vi "Get All Sub-vis in Heirarchy.vi"(8 "error in (no error)":errorcluster, 11 "Start Vi":refnum<vi>) -> (0 "error out":errorcluster, 2 "All sub-vi nodes in heirarchy":refnum<vi>[](array[refnum]), 3 "Start Vi out":refnum<vi>, 4 "Vi Names":string[](array[string]), 5 "Vi-Refs":refnum<vi>[](array[refnum]))   [LabVIEW 2012, in "Scripting Tools.lvlib"]
doc: "Returns all the sub-vi nodes in all the diagrams of all the vis in the heirarchy, starting from <b>Start Vi</b>. Also returns a list of references to the vis (as opposed to the sub-vi nodes) and to the vi names."
uses:
  Scripting Tools.lvlib
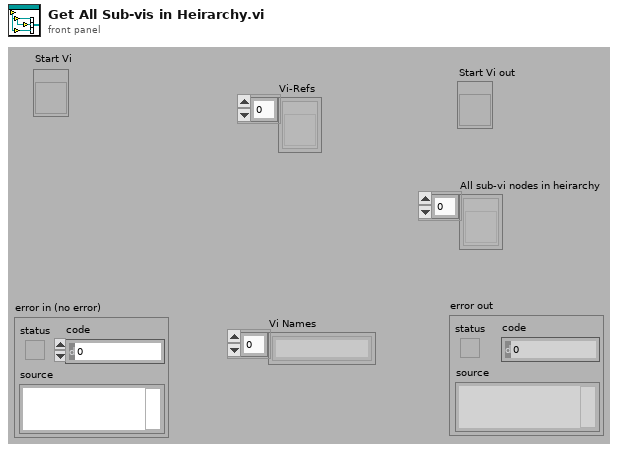
[diagram p1: front panel]
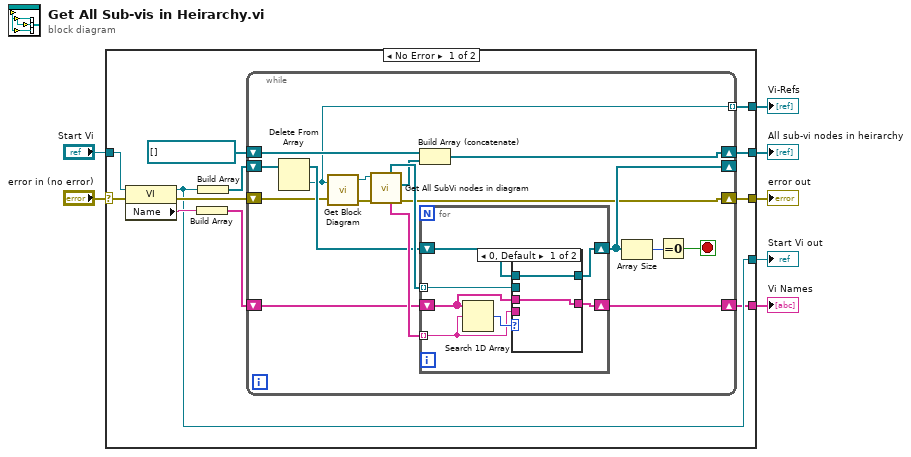
[diagram p0: block diagram]
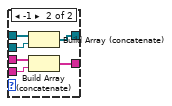
[diagram p2: hidden frame]
diagram:
  n1 = case shown="No Error" "error in (no error)" {
    selector: "error in (no error)" -> [w11 w53]
    tunnel: "Start Vi" -> [w17 w52]
    tunnel: [w14 _] -> w6
    tunnel: [w12 w53] -> w5
    tunnel: [w10 w52] -> w3
    tunnel: [w9 _] -> w2
    tunnel: [w8 _] -> w1
    frame No Error {
      n2 = property class="VI"(reference=w17, error in=w11) -> (reference out=w10:refnum<vi>, error out=w13:errorcluster, "Name"=w16:string)
      n3 = Build Array(w16) -> (w18:string[])
      n4 = Build Array(w10) -> (w19:refnum<vi>[])
      n5 = while {
        shift-right: [w24] -> w14
        shift-left: refnum<vi>[] [] -> [w23]
        shift-right: [w28] -> _
        shift-left: w19 -> [w36]
        shift-right: [w29] -> w8
        shift-left: w18 -> [w31]
        shift-right: [w21] -> w12
        shift-left: w13 -> [w22]
        tunnel: [w20] -> w9 mode=indexing
        stop <- w26 stop-if-true
        n6 = Delete From Array(array=w36) -> (deleted portion=w20:refnum<vi>, array with subset deleted=w30:refnum<vi>[])  [unwired: 2 in]
        n7 = call "Get Block Diagram.vi"("vi refnum in"=w20, "error in (no error)"=w22) -> ("Diagram"=w35:refnum<vi>, "error out"=w34:errorcluster)  [unwired: 1 out]
        n8 = call "Get All SubVi nodes in diagram.vi"("error in"=w34, "Diagram In"=w35) -> ("error out"=w21:errorcluster, "All Sub-vis"=w25:refnum<vi>[], "Vi Names"=w32:string[], "Vi-Refs"=w33:refnum<vi>[])  [unwired: 6 out]
        n9 = Build Array (concatenate)(w23, w25) -> (w24:refnum<vi>[])
        n10 = for {
          tunnel: w33 -> [w37] mode=indexing
          tunnel: w32 -> [w41] mode=indexing
          shift-right: [w40] -> w29
          shift-left: w31 -> [w42]
          shift-right: [w38] -> w28
          shift-left: w30 -> [w39]
          n11 = Search 1D Array(1D array=w42, element=w41) -> (index of element=w43:i32)  [unwired: 1 out]
          n12 = case shown="0, Default" w43 {
            tunnel: w42 -> [w45 w49]
            tunnel: w41 -> [_ w51]
            tunnel: [w45 w50] -> w40
            tunnel: w39 -> [w44 w48]
            tunnel: [w44 w47] -> w38
            tunnel: w37 -> [_ w46]
            frame 0, Default {
            }
            frame -1 {
              n13 = Build Array (concatenate)(w48, w46) -> (w47:refnum<vi>[])
              n14 = Build Array (concatenate)(w49, w51) -> (w50:string[])
            }
          }
        }
        n15 = Array Size(array=w28) -> (size(s)=w27:i32)
        n16 = Equal To 0?(x=w27) -> (x = 0?=w26:bool)
      }
    }
    frame Error {
    }
  }
  "All sub-vi nodes in heirarchy" <- w6
  "error out" <- w5
  "Start Vi out" <- w3
  "Vi-Refs" <- w2
  "Vi Names" <- w1
